vi "Brickwall_LowPass.vi"(7 "Max Freq":dbl, 9 "time signal":waveform(dbl)) -> (1 "output waveform":waveform(dbl), 2 "output Phase":cluster{"f0":dbl, "df":dbl, "phase":dbl[]}, 3 "output Mag":cluster{"f0":dbl, "df":dbl, "magnitude":dbl[]}, 10 "phase":cluster{"f0":dbl, "df":dbl, "phase":dbl[]} {"phase" format="%.2p"; "f0" format="%0.2p"; "df" format="%0.2p"}, 11 "magnitude":cluster{"f0":dbl, "df":dbl, "magnitude":dbl[]} {"magnitude" format="%.2p"; "f0" format="%0.2p"; "df" format="%0.2p"})   [LabVIEW 2021]
uses:
  <vilib>/Analysis/4window.llb/windowTd.ctl
  <vilib>/Analysis/2dsp.llb/Inverse Real FFT.vi
  <vilib>/measure/maspectr.llb/FFT Spectrum (Mag-Phase) for 1 Chan.vi
  <vilib>/measure/NI_MAPro.lvlib
  <vilib>/Analysis/NI_AALPro.lvlib
panel:
  out "Waveform Graph 2":waveform(dbl)[](graph)
  out "Waveform Graph":cluster{"f0":dbl, "df":dbl, "magnitude":dbl[]}[](graph)
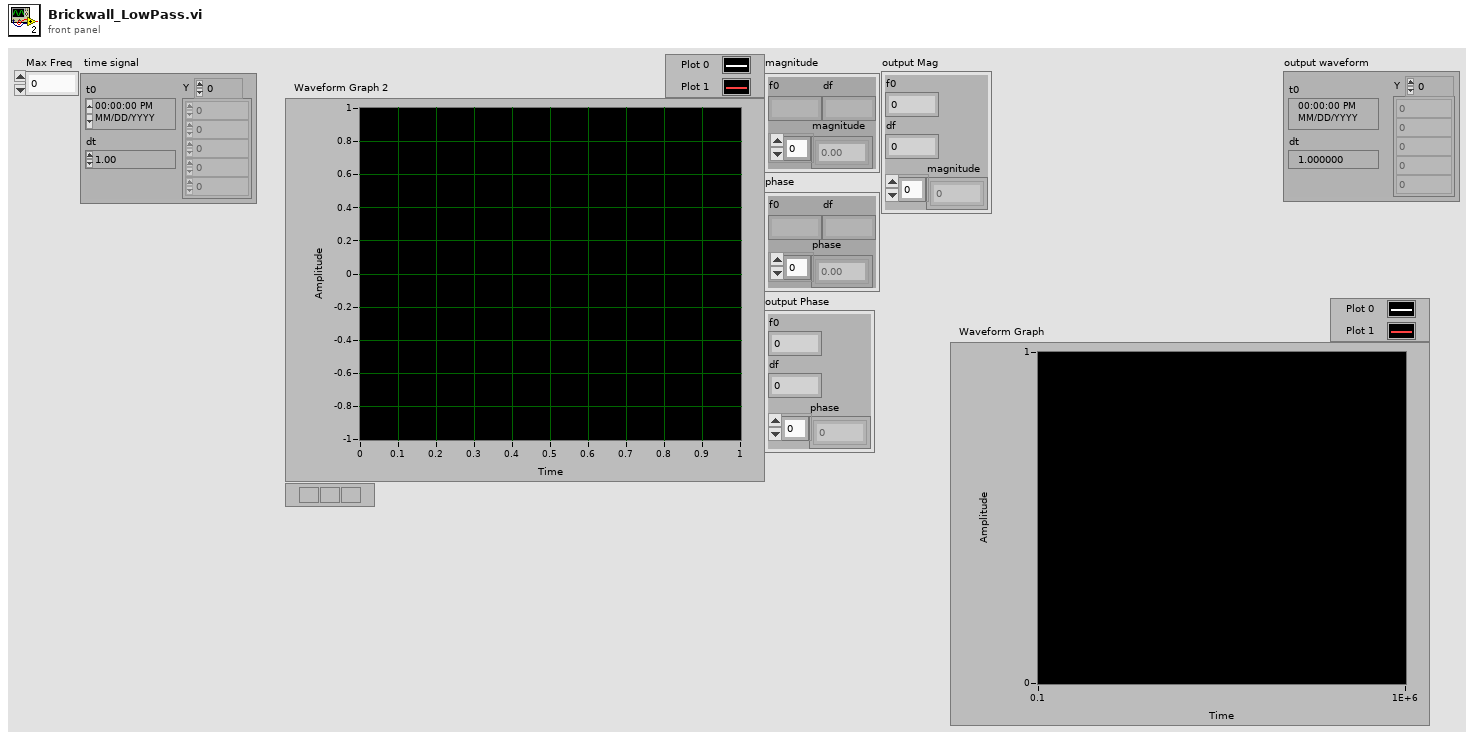
[diagram p1: front panel]
types:
  T1 = typedef "NI_AALPro.lvlib/windowTd.ctl" = u32
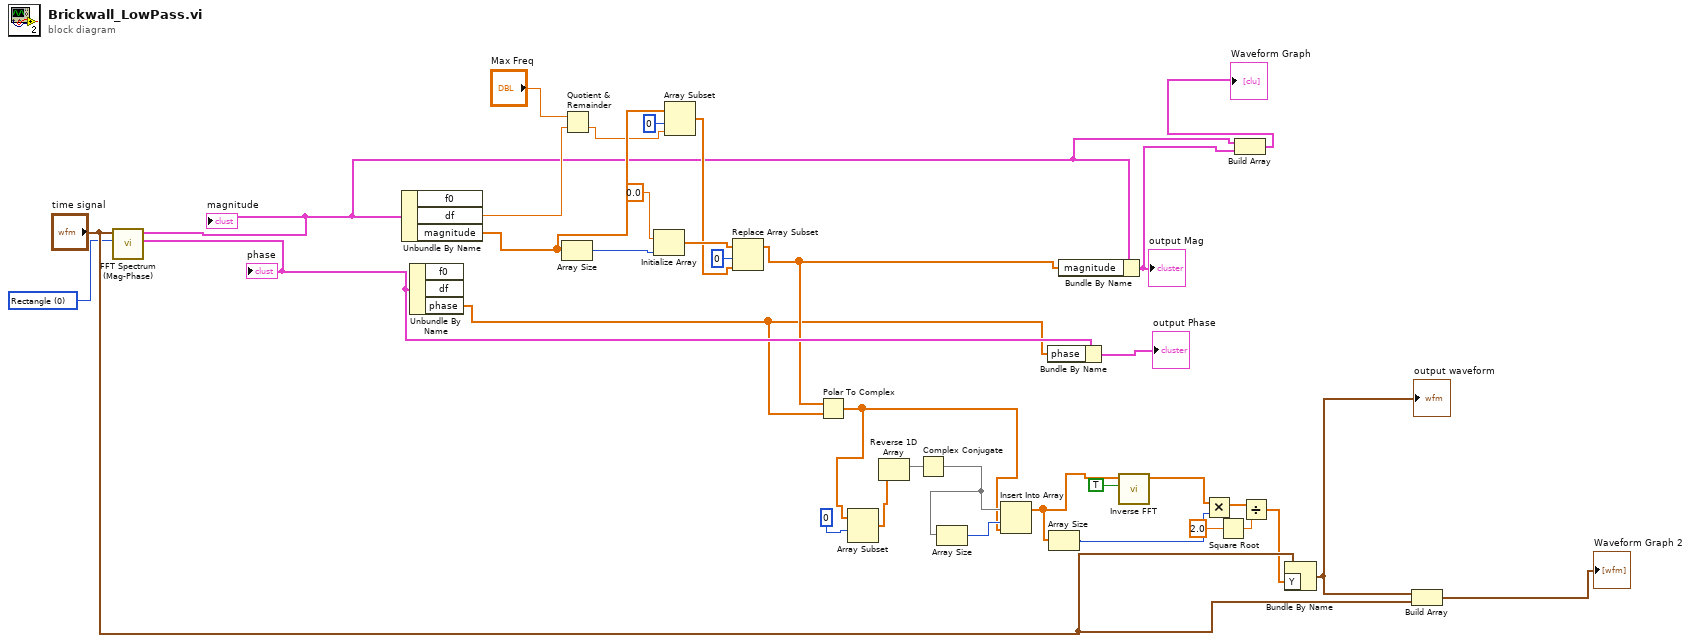
[diagram p0: block diagram]
diagram:
  w15 = T1 0 items=["Rectangle"=0, "Hanning"=1, "Hamming"=2, "Blackman-Harris"=3, "Exact Blackman"=4, "Blackman"=5, "Flat Top"=6, "4 Term B-Harris "=7, "7 Term B-Harris"=8, "Low Sidelobe"=9, "Blackman Nuttall"=11, "Triangle"=30, "Bartlett-Hanning"=31, "Bohman"=32, "Parzen"=33, "Welch"=34, "Kaiser"=60, "Dolph-Chebyshev"=61, "Gaussian"=62] ("window")
  n1 = call-poly <vilib>:"FFT Spectrum (Mag-Phase).vi"("window"=w15, "time signal"="time signal") -> ("phase"=w21:cluster{"f0":dbl, "df":dbl, "phase":dbl[]}, "magnitude"=w22:cluster{"f0":dbl, "df":dbl, "magnitude":dbl[]})  [unwired: 5 in, 3 out]
  "magnitude" <- w22
  "phase" <- w21
  n2 = Unbundle By Name(w22) -> ("df"=w31:dbl, "magnitude"=w30:dbl[])  [unwired: 1 out]
  n3 = Unbundle By Name(w21) -> ("phase"=w19:dbl[])  [unwired: 2 out]
  n4 = Array Size(array=w30) -> (size(s)=w35:i32)
  n5 = Quotient & Remainder(x="Max Freq", y=w31) -> (floor(x/y)=w28:dbl)  [unwired: 1 out]
  n6 = Initialize Array(0.0 ("element"), w35) -> (w33:dbl[])
  n7 = Array Subset(array=w30, index=0, length=w28) -> (w26:dbl[])
  n8 = Replace Array Subset(array=w33, new element=w26, index=0) -> (w20:dbl[])
  n9 = Polar To Complex(1:w19, 2:w20) -> (0:w9:cdb[])
  n10 = Array Subset(array=w9, index=0) -> (w7:cdb[])  [unwired: 1 in]
  n11 = Reverse 1D Array(array=w7) -> (reversed array=w14:cdb[])
  n12 = Complex Conjugate(1:w14) -> (0:w12:cdb[])
  n13 = Array Size(array=w12) -> (size(s)=w11:i32)
  n14 = Insert Into Array(array=w12, index=w11, new element=w9) -> (w5:cdb[])
  n15 = Bundle By Name(cluster=w21, "phase"=w19) -> (→"output Phase":cluster{"f0":dbl, "df":dbl, "phase":dbl[]})
  n16 = Array Size(array=w5) -> (size(s)=w10:i32)
  n17 = Bundle By Name(cluster=w22, "magnitude"=w20) -> (w24:cluster{"f0":dbl, "df":dbl, "magnitude":dbl[]})
  "output Mag" <- w24
  n18 = call-poly <vilib>:"Inverse FFT.vi"("shift?"=TRUE, "FFT {X}"=w5) -> ("X"=w13:dbl[])  [unwired: 8 in, 1 out]
  n19 = Multiply(x=w13, y=w10) -> (x*y=w4:dbl[])
  n20 = Square Root(x=2.0) -> (sqrt(x)=w2:dbl)
  n21 = Build Array(w22, w24) -> (→"Waveform Graph":cluster{"f0":dbl, "df":dbl, "magnitude":dbl[]}[])
  n22 = Divide(x=w4, y=w2) -> (x/y=w3:dbl[])
  n23 = Bundle By Name(cluster="time signal", "Y"=w3) -> (w18:waveform(dbl))
  "output waveform" <- w18
  n24 = Build Array(w18, "time signal") -> (→"Waveform Graph 2":waveform(dbl)[])
